vi "InitDL.vi"(3 "Container State":T4 caption="État du conteneur", 4 "Previous State":variant caption="État précédent", 5 "Previous Version":T3 caption="Version précédente") -> (2 "Current State":T1={"param"={"Short"={"min"=-100.0, "max"=48.0, "real pos"=-48.0}, "Long"={"min"=-900.0, "max"=100.0, "real pos"=-100.0}}, "pos short"=0.0, "pos long"=0.0, "DL short"=refnum, "DL long"=refnum, "Cells"=enum."7", "cell pos"=[]} caption="État actuel")   [LabVIEW 2015, in "ControlDL.xctl"]
uses:
  ControlDL.xctl
  stateDL.ctl
  controls/CellsSD.ctl
  controls/CellBoolean.ctl
  <vilib>/_xctls/Container State.ctl
  <vilib>/_xctls/Version.ctl
  <vilib>/_xctls/XControlSupport.lvlib
panel:
  in  "Default Indicator State":T1={"param"={"Short"={"min"=-100.0, "max"=48.0, "real pos"=-48.0}, "Long"={"min"=-900.0, "max"=100.0, "real pos"=-100.0}}, "pos short"=0.0, "pos long"=0.0, "DL short"=refnum, "DL long"=refnum, "Cells"=enum."7", "cell pos"=[]} caption="État de l'indicateur par défaut"
  in  "Default Control State":T1={"param"={"Short"={"min"=-100.0, "max"=48.0, "real pos"=-48.0}, "Long"={"min"=-900.0, "max"=100.0, "real pos"=-100.0}}, "pos short"=0.0, "pos long"=0.0, "DL short"=refnum, "DL long"=refnum, "Cells"=enum."7", "cell pos"=[]} caption="État de la commande par défaut"
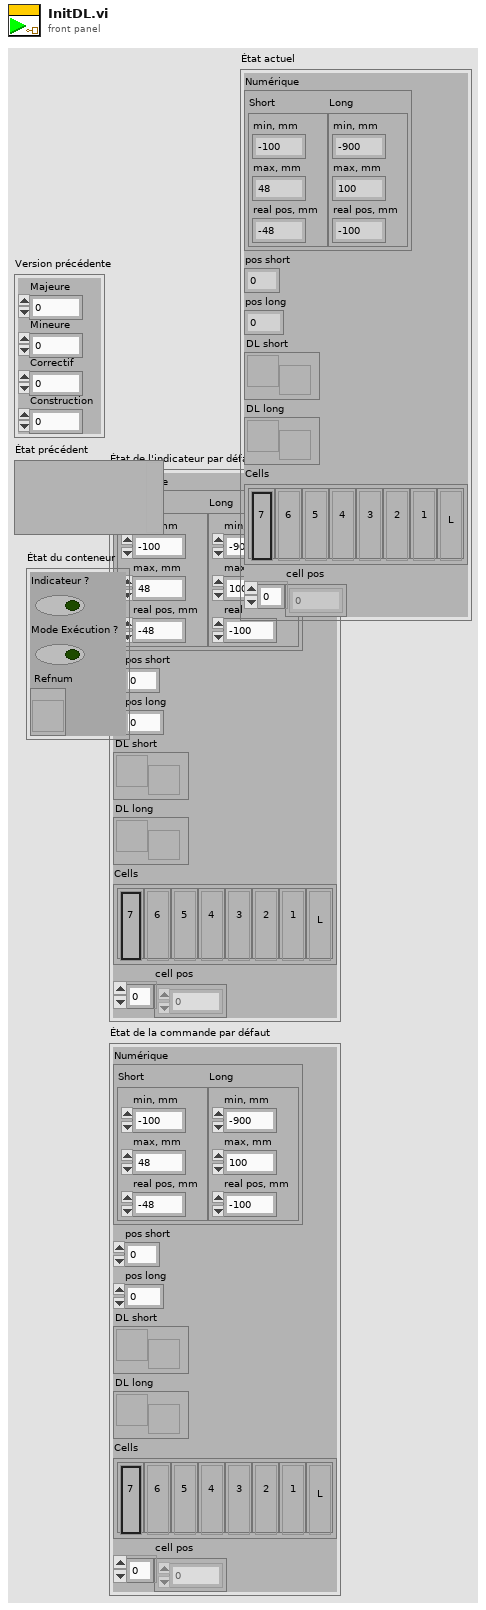
[diagram p1: front panel]
types:
  T1 = typedef "ControlDL.xctl/stateDL.ctl" = cluster{"param":cluster{"Short":cluster{"min":dbl, "max":dbl, "real pos":dbl}, "Long":cluster{"min":dbl, "max":dbl, "real pos":dbl}}, "pos short":dbl, "pos long":dbl, "DL short":refnum<user-event>, "DL long":refnum<user-event>, "Cells":T2, "cell pos":dbl[]}
  T2 = typedef "CellsSD.ctl" = enum32{"7", "6", "5", "4", "3", "2", "1", "L"}
  T3 = typedef "XControlSupport.lvlib/Version.ctl" = cluster{"Major":u16, "Minor":u16, "Fix":u16, "Build":u16}
  T4 = typedef "XControlSupport.lvlib/Container State.ctl" = cluster{"Indicator?":bool, "Run Mode?":bool, " Refnum":refnum<vi>}
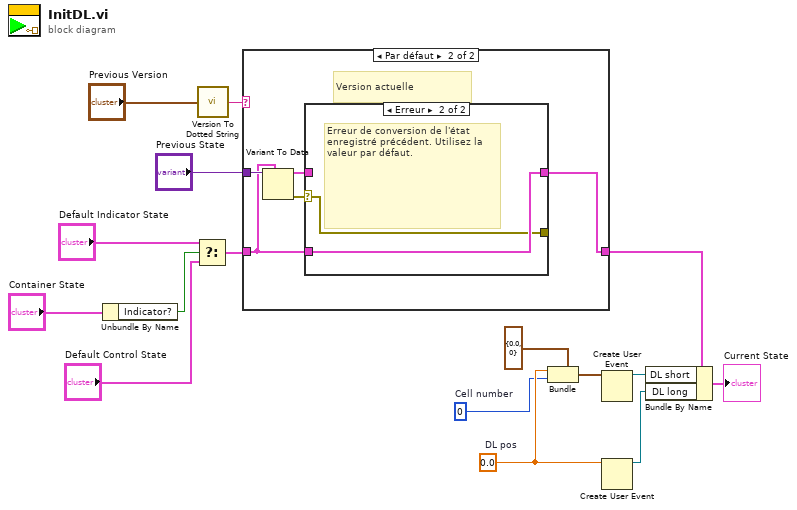
[diagram p0: block diagram]
diagram:
  w4 = 0  # Cell number
  w5 = 0.0  # DL pos
  n1 = Unbundle By Name("Container State") -> ("Indicator?"=w12:bool)
  n2 = Select(t="Default Indicator State", s=w12, f="Default Control State") -> (s? t:f=w11:T1)
  n3 = call <vilib>:"Version To Dotted String.vi"("Version"="Previous Version") -> ("String Version"=w9:string)
  n4 = case shown="Par défaut" w9 {
    tunnel: "Previous State" -> [_ w22]
    tunnel: [w17 w18] -> w8
    tunnel: w11 -> [w17 w19]
    frame "0.0.0.0" {
      # "Nouvelle création ; utilisez l'état par défaut"
    }
    frame Default {
      # "Version actuelle"
      n5 = Variant To Data(type=w19, Variant=w22) -> (data=w20:T1, error out=w21:errorcluster)  [unwired: 1 in]
      n6 = case shown="Erreur" w21 {
        selector: w21 -> [w24 w25]
        tunnel: w20 -> [w23 _]
        tunnel: [w23 w26] -> w18
        tunnel: w19 -> [_ w26]
        tunnel: [w24 w25] -> _
        frame No Error {
        }
        frame Error {
          # "Erreur de conversion de l'état\nenregistré précédent. Utilisez la valeur par défaut."
        }
      }
    }
  }
  n7 = Bundle(cluster=cluster{"DL pos":dbl, "Cell number":i32} {"DL pos"=0.0, "Cell number"=0} ("output cluster"), "DL pos"=w5, "Cell number"=w4) -> (w3:cluster{"DL pos":dbl, "Cell number":i32})
  n8 = Create User Event(user event datatype=w3) -> (user event=w1:refnum<user-event>)  [unwired: 1 in, 1 out]
  n9 = Create User Event(user event datatype=w5) -> (user event=w6:refnum<user-event>)  [unwired: 1 in, 1 out]
  n10 = Bundle By Name(cluster=w8, "DL short"=w1, "DL long"=w6) -> (→"Current State":T1)
